vi "calc exptime diff.vi"(8 "error in (no error)":errorcluster, 10 "ACS mode":bool, 11 "Simulated_CCD_Camera in":refnum<class "Simulated_CCD_Camera.lvclass">) -> (0 "error out":errorcluster, 2 "error out":errorcluster, 3 "Simulated_CCD_Camera out":refnum<class "Simulated_CCD_Camera.lvclass">)   [LabVIEW 2018, in "Simulated_CCD_Camera.lvclass"]
uses:
  Simulated_CCD_Camera.lvclass
  Simulated_CCD_Camera.lvclass/Simulated_CCD_Camera.ctl
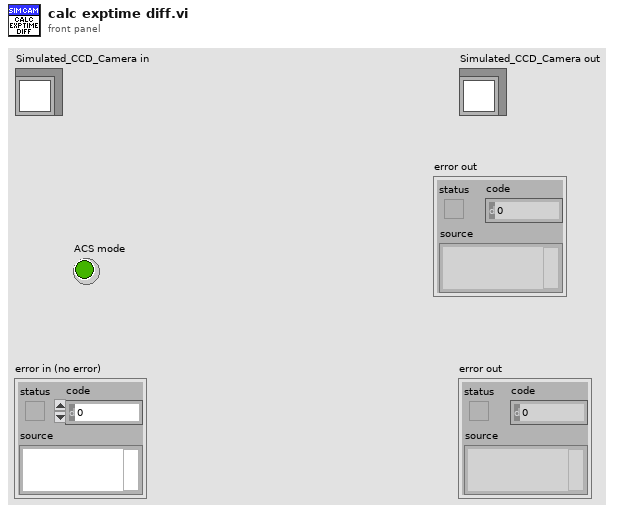
[diagram p1: front panel]
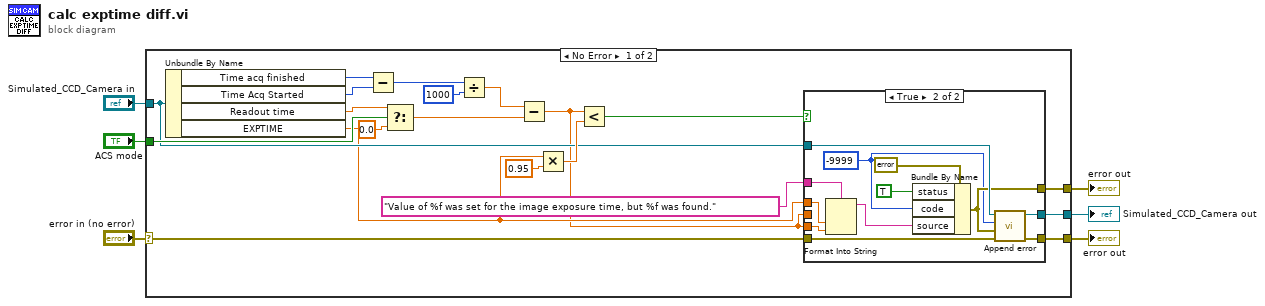
[diagram p0: block diagram]
diagram:
  n1 = case shown="No Error" "error in (no error)" {
    selector: "error in (no error)" -> [w14 w42]
    tunnel: [w12 w42] -> w5
    tunnel: [w13 w41] -> w3
    tunnel: "Simulated_CCD_Camera in" -> [w15 w41]
    tunnel: "ACS mode" -> [w16 _]
    tunnel: [w10 _] -> w1
    frame No Error {
      n2 = Unbundle By Name(w15) -> ("Time acq finished"=w26:u32, "Time Acq Started"=w25:u32, "Readout time"=w19:dbl, "EXPTIME"=w9:dbl)
      n3 = Subtract(x=w26, y=w25) -> (x-y=w22:u32)
      n4 = Select(t=w19, s=w16, f=0.0) -> (s? t:f=w17:dbl)
      n5 = Divide(x=w22, y=1000) -> (x/y=w20:dbl)
      n6 = Subtract(x=w20, y=w17) -> (x-y=w8:dbl)
      n7 = Multiply(x=w9, y=0.95) -> (x*y=w24:dbl)
      n8 = Less?(x=w8, y=w24) -> (x < y?=w11:bool)
      n9 = case shown="True" w11 {
        tunnel: w8 -> [_ _]
        tunnel: w15 -> [w27 w35]
        tunnel: w14 -> [w28 w37]
        tunnel: [w27 w34] -> w13
        tunnel: [w28 w36] -> w12
        tunnel: [_ w33] -> w10
        tunnel: w9 -> [_ w31]
        tunnel: w8 -> [_ w30]
        tunnel: "Value of %f was set for the image exposure time, but %f was found." -> [_ w29]
        frame False {
        }
        frame True {
          w32 = -9999 ("code")
          n10 = Format Into String(format string=w29, w31, w30) -> (resulting string=w38:string)  [unwired: 2 in, 1 out]
          n11 = Bundle By Name(cluster=errorcluster {"status"=FALSE, "code"=0, "source"=""} ("error out 2"), "status"=TRUE, "code"=w32, "source"=w38) -> (w33:errorcluster)
          n12 = call "Append error.vi"("error in (no error)"=w37, "error"=w33, "code"=w32, "Simulated_CCD_Camera in"=w35) -> ("error out"=w36:errorcluster, "Simulated_CCD_Camera out"=w34:refnum<class "Simulated_CCD_Camera.lvclass">)  [unwired: 6 in]
        }
      }
    }
    frame Error {
    }
  }
  "error out" <- w5
  "Simulated_CCD_Camera out" <- w3
  "error out" <- w1
